vi "CR-衬丝检测处理函数.vi"(0 "Image in":T9(plugin-control), 5 "CR- 衬丝检测参数":T8={"Settings (Clamp (Rake) 1)"={"Contrast"=65, "Filter width"=3, "Steepness"=6, "Subsampling Ratio"=9, "Show Search Area"=TRUE, "Show Search Lines"=FALSE, "Show Edges Found"=FALSE, "Show Result"=TRUE}, "Options (Find Straight Edge 1)"={"Search Direction"=0, "Edge Options"={"Edge Polarity"=1, "Kernel Size"=13, "Width"=1, "Minimum Edge Strength"=25.0, "Interpolation Type"=enum."Bilinear Fixed", "Data Processing Method"=enum."Average"}, "Show Search Area"=FALSE, "Show Search Lines"=FALSE, "Show Edges Found"=FALSE, "Show Result"=FALSE, "Search Area Color"=65280, "Search Lines Color"=255, "Edge Locations Color"=16776960, "Result Color"=16711680, "Overlay Group Name"=""}, "相对距离设定"={"上限"=925.0, "下限"=3.0}, "保护套角度"={"上限"=0.0, "下限"=0.0}, "保护套直径设定"={"上限"=0.0, "下限"=0.0}, "Edge Options (Edge Detector 1)"={"Edge Polarity"=0, "Kernel Size"=3, "Width"=3, "Minimum Edge Strength"=10.0, "Interpolation Type"=enum."Bilinear Fixed", "Data Processing Method"=enum."Average"}, "保护套标准位置"={"Start X"=0, "Start Y"=0, "End X"=0, "End Y"=0}} {"保护套标准位置"."Start X" scale=0.0..1024.0; "保护套标准位置"."End X" scale=0.0..1024.0; "Edge Options (Edge Detector 1)"."Edge Polarity" items=["All Edges", "Rising Edges", "Falling Edges"]; "Options (Find Straight Edge 1)"."Search Direction" items=["Left to Right", "Right to Left", "Top to Bottom", "Bottom to Top"]; "Options (Find Straight Edge 1)"."Edge Options"."Edge Polarity" items=["All Edges", "Rising Edges", "Falling Edges"]; "Options (Find Straight Edge 1)"."Edge Options"."Minimum Edge Strength" format="%.2f"; "Options (Find Straight Edge 1)"."Edge Options"."Width" step=2; "Options (Find Straight Edge 1)"."Edge Options"."Kernel Size" step=2}, 7 "CR- 衬丝检测ROI参数":T4 {"Line 2"."Start X" scale=0.0..1024.0; "Line 2"."End X" scale=0.0..1024.0; "clamp Rectangle"."Rotation" min=-90.0 max=90.0 step=1.0 format="%.2f"; "clamp Rectangle"."Left" scale=0.0..1024.0; "clamp Rectangle"."Right" scale=0.0..1024.0; "Line 1"."Start X" scale=0.0..1024.0; "Line 1"."End X" scale=0.0..1024.0; "find straight edge Rectangle"."Rotation" min=-90.0 max=90.0 step=1.0 format="%.2f"; "find straight edge Rectangle"."Left" scale=0.0..1024.0; "find straight edge Rectangle"."Right" scale=0.0..1024.0}, 11 "error in (no error)":errorcluster caption="错误输入（无错误）") -> (4 "Image out":T9(plugin-control), 6 "Distance (Clamp (Rake) 1)":sgl format="%.2f", 8 "保护套距离":bool, 10 "衬丝有无":bool, 13 "保护套直径":sgl, 14 "保护套与基准位置差值":sgl, 15 "error out":errorcluster caption="错误输出")   [LabVIEW 2017]
uses:
  <vilib>/vision/Measure.llb/Edge Options.ctl
  <vilib>/vision/Measure.llb/Edge Polarity.ctl
  <vilib>/vision/Measure.llb/Edge New.ctl
  <vilib>/vision/NI_Vision_Development_Module.lvlib
panel:
  in  "Settings (Clamp (Rake) 1)":T1={"Contrast"=66, "Filter width"=8, "Steepness"=11, "Subsampling Ratio"=7, "Show Search Area"=TRUE, "Show Search Lines"=TRUE, "Show Edges Found"=TRUE, "Show Result"=TRUE}
  out "Angle (Real-World)":dbl
  out "保护套与基准位置差值":bool
  out "Location (Real-World)":cluster{"X":sgl, "Y":sgl}
  out "Edge Information (Edge Detector 2)":T5[](array[typedef]) {"Distance (Real-World)" format="%.2f"; "Location (Real-World)"."Y" format="%.2g"; "Location (Real-World)"."X" format="%.2f"; "Noise" format="%.2f"; "Location (Pixel)"."Y" format="%.2g"; "Location (Pixel)"."X" format="%.2f"; "Strength" format="%.2f"; "Distance (Pixel)" format="%.2f"}
  out "Edge Information (Edge Detector 1)":T5[](array[typedef]) {"Distance (Real-World)" format="%.2f"; "Location (Real-World)"."Y" format="%.2g"; "Location (Real-World)"."X" format="%.2f"; "Noise" format="%.2f"; "Location (Pixel)"."Y" format="%.2g"; "Location (Pixel)"."X" format="%.2f"; "Strength" format="%.2f"; "Distance (Pixel)" format="%.2f"}
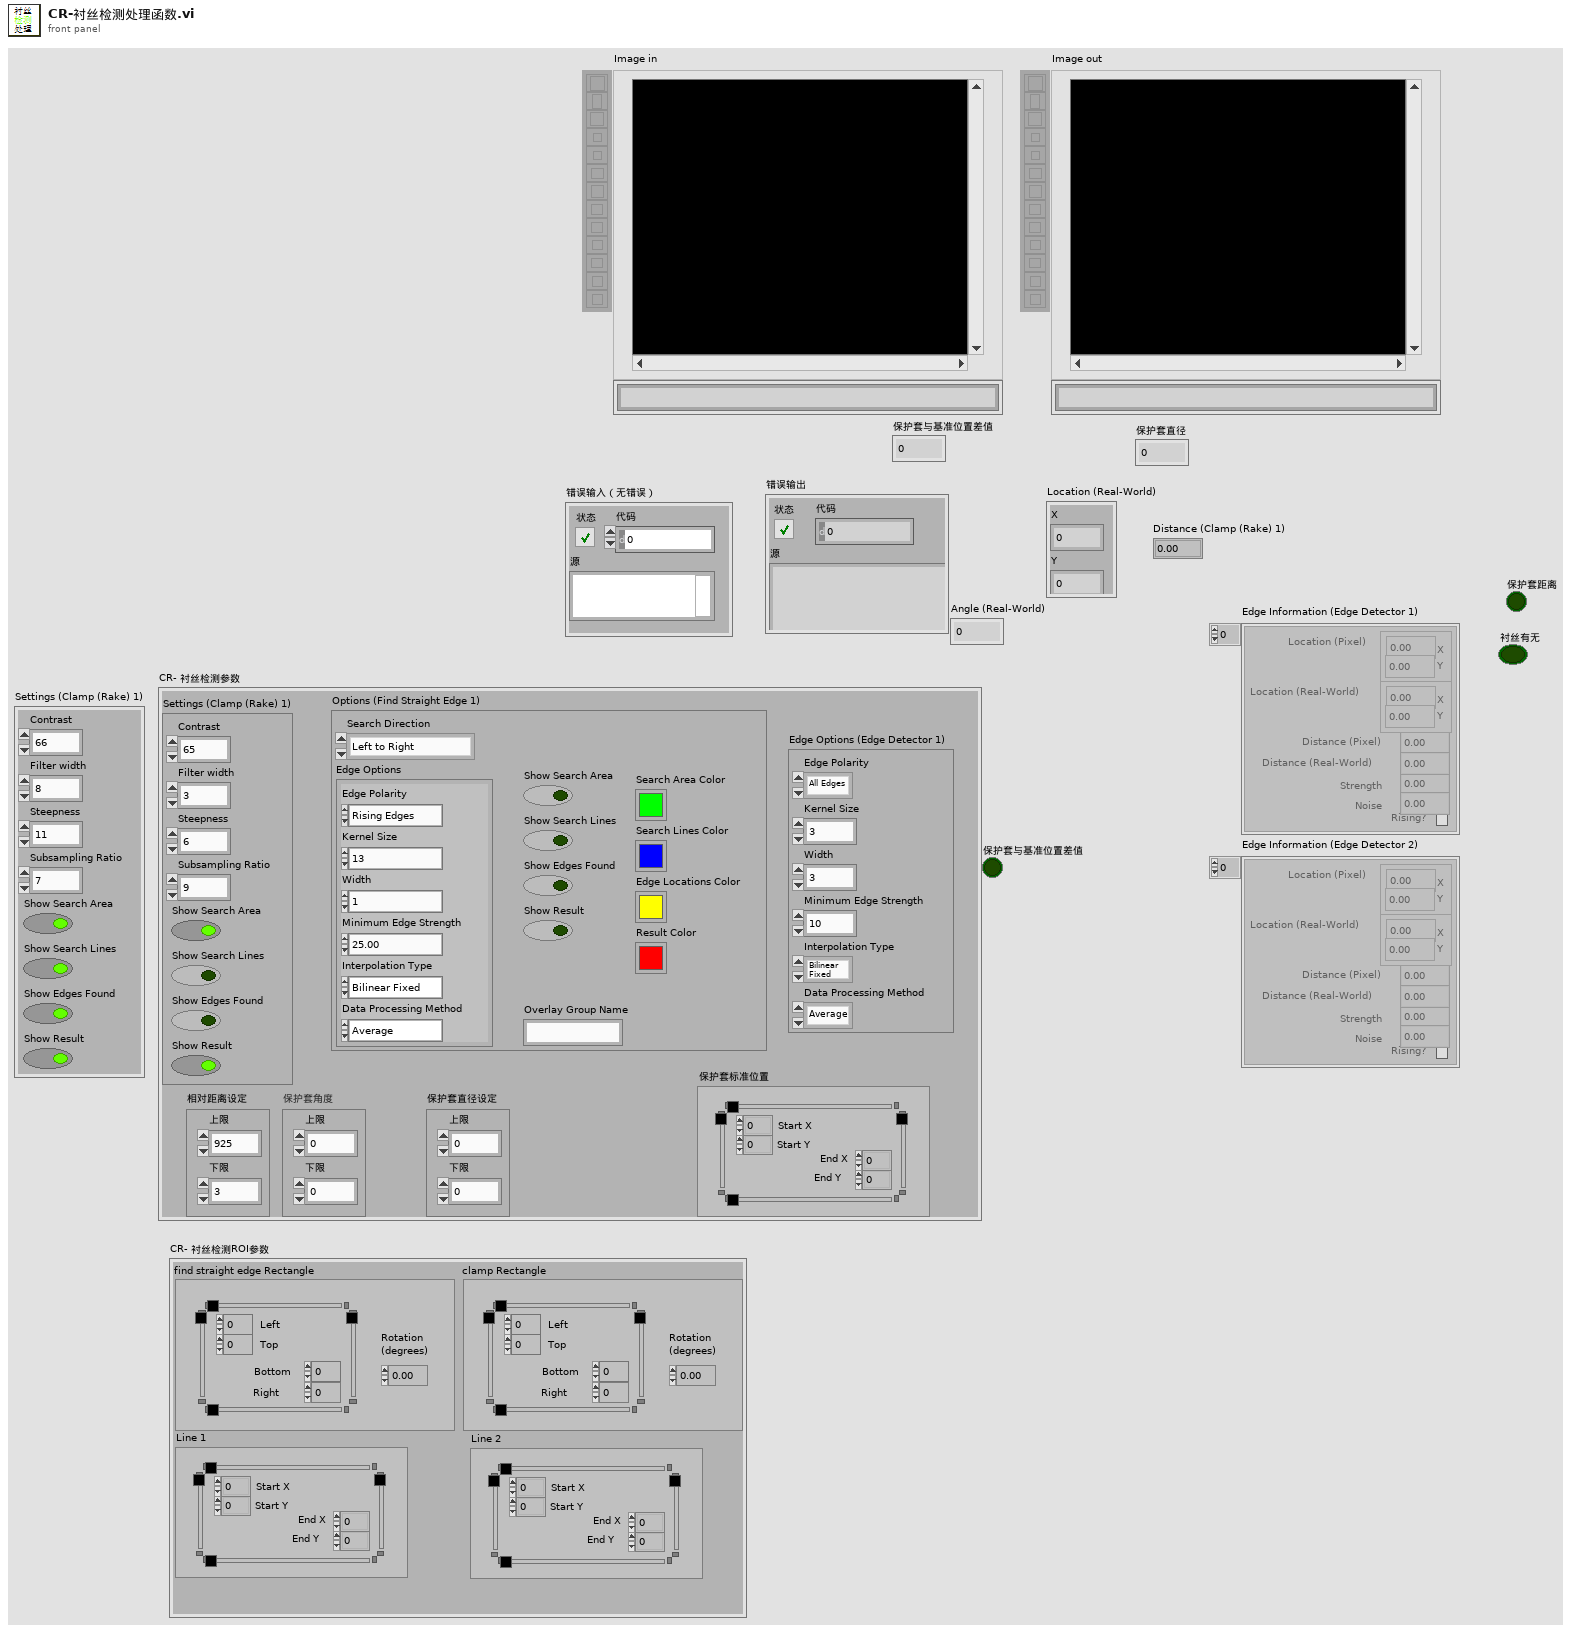
[diagram p1: front panel]
types:
  T1 = cluster{"Contrast":i32, "Filter width":i32, "Steepness":i32, "Subsampling Ratio":u32, "Show Search Area":bool, "Show Search Lines":bool, "Show Edges Found":bool, "Show Result":bool}
  T2 = typedef "IMAQ Rectangle" = cluster{"Left":i32, "Top":i32, "Right":i32, "Bottom":i32, "Rotation":dbl}
  T3 = typedef "IMAQ Line" = cluster{"Start X":i32, "Start Y":i32, "End X":i32, "End Y":i32}
  T4 = cluster{"find straight edge Rectangle":T2, "Line 1":T3, "clamp Rectangle ":T2, "Line 2":T3}
  T5 = typedef "Edge New.ctl" = cluster{"Location (Pixel)":cluster{"X":sgl, "Y":sgl}, "Location (Real-World)":cluster{"X":sgl, "Y":sgl}, "Distance (Pixel)":dbl, "Distance (Real-World)":dbl, "Strength":dbl, "Noise":dbl, "Rising?":bool}
  T6 = typedef "Edge Options.ctl" = cluster{"Edge Polarity":T7, "Kernel Size":u32, "Width":u32, "Minimum Edge Strength":sgl, "Interpolation Type":enum32{"Zero Order", "Bilinear", "Quadratic", "Cubic", "Bilinear Fixed"}, "Data Processing Method":enum32{"Average", "Median"}}
  T7 = typedef "Edge Polarity.ctl" = u32
  T8 = cluster{"Settings (Clamp (Rake) 1)":cluster{"Contrast":i32, "Filter width":i32, "Steepness":i32, "Subsampling Ratio":u32, "Show Search Area":bool, "Show Search Lines":bool, "Show Edges Found":bool, "Show Result":bool}, "Options (Find Straight Edge 1)":cluster{"Search Direction":u32, "Edge Options":T6, "Show Search Area":bool, "Show Search Lines":bool, "Show Edges Found":bool, "Show Result":bool, "Search Area Color":u32, "Search Lines Color":u32, "Edge Locations Color":u32, "Result Color":u32, "Overlay Group Name":string}, "相对距离设定":cluster{"上限":dbl, "下限":dbl}, "保护套角度":cluster{"上限":dbl, "下限":dbl}, "保护套直径设定":cluster{"上限":dbl, "下限":dbl}, "Edge Options (Edge Detector 1)":cluster{"Edge Polarity":u32, "Kernel Size":u32, "Width":u32, "Minimum Edge Strength":sgl, "Interpolation Type":enum32{"Zero Order", "Bilinear", "Quadratic", "Cubic", "Bilinear Fixed"}, "Data Processing Method":enum32{"Average", "Median"}}, "保护套标准位置":T3}
  T9 = typedef "IMAQ Image.ctl" = refnum<image>
  T10 = cluster{"Search Direction":u32, "Edge Options":T6, "Show Search Area":bool, "Show Search Lines":bool, "Show Edges Found":bool, "Show Result":bool, "Search Area Color":u32, "Search Lines Color":u32, "Edge Locations Color":u32, "Result Color":u32, "Overlay Group Name":string}
  T11 = cluster{"Global Rectangle":i32[], "Contours":cluster{"ID":enum32{"External", "Internal"}, "Type":u32, "Coordinates":i32[]}[]}
  T12 = cluster{"Desired Font (Application)":enum16{"User-specified Font", "Application Font", "System Font", "Dialog Font"}, "[User-specified Font]":cluster{"Font Name":string, "Size":i16, "Strikeout?":bool, "Italic?":bool, "Underline?":bool, "Outline?":bool, "Shadow?":bool, "Bold?":bool, "Rotation Angle":dbl}, "Horizontal Alignment":i16, "Vertical Alignment":i16}
  T13 = typedef "ROI Descriptor" = cluster{"Global Rectangle":i32[], "Contours":cluster{"ID":enum32{"External", "Internal"}, "Type":u32, "Coordinates":i32[]}[]}
  T14 = cluster{"Point1 (Pixels)":cluster{"X":sgl, "Y":sgl}, "Point2 (Pixels)":cluster{"X":sgl, "Y":sgl}, "Point1 (Real-World)":cluster{"X":sgl, "Y":sgl}, "Point2 (Real-World)":cluster{"X":sgl, "Y":sgl}, "Angle (Pixel)":dbl, "Angle (Real-World)":dbl, "Score":dbl, "Straightness":dbl, "Average SNR (db)":dbl, "Calibration Valid":bool}
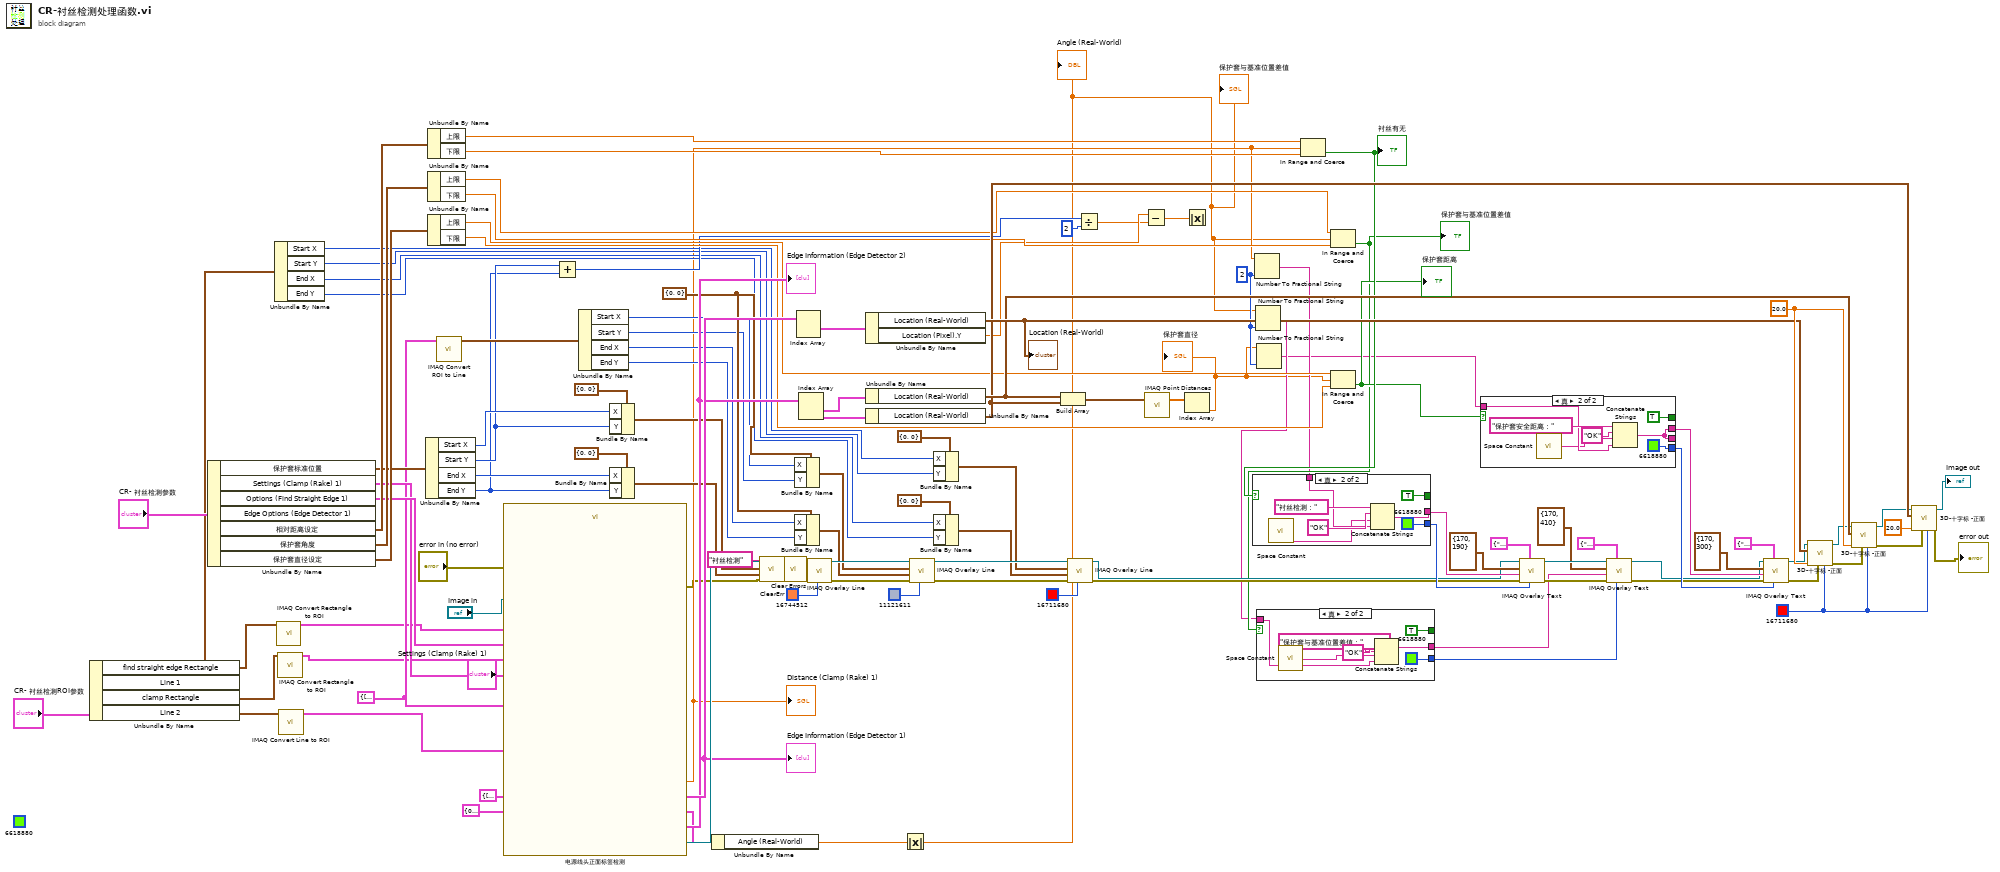
[diagram p0: block diagram]
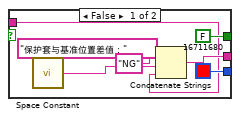
[diagram p2: hidden frame]
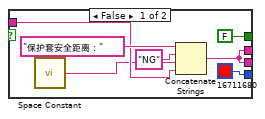
[diagram p3: hidden frame]
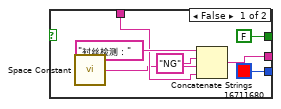
[diagram p4: hidden frame]
diagram:
  w15 = i16 2 ("精度(6)")
  w68 = cluster{"X":i32, "Y":i32} {"X"=0, "Y"=0} ("Start Point")
  w73 = T11 {"Global Rectangle"=[1263, 312, 1264, 1097], "Contours"=[{"ID"=enum."External", "Type"=2, "Coordinates"=[1263, 312, 1263, 1096]}]} ("ROI Descriptor (保护套位置)")
  (unwired) u32 6618880 ("Color")
  w105 = u32 16711680 ("Color")
  w107 = 20.0 ("radius")
  n1 = Unbundle By Name("CR- 衬丝检测ROI参数") -> ("find straight edge Rectangle"=w33:T2, "clamp Rectangle"=w32:T2, "Line 2"=w42:T3)  [unwired: 1 out]
  n2 = Unbundle By Name("CR- 衬丝检测参数") -> ("保护套标准位置"=w82:T3, "Settings (Clamp (Rake) 1)"=w84:T1, "Options (Find Straight Edge 1)"=w85:T10, "相对距离设定"=w98:cluster{"上限":dbl, "下限":dbl}, "保护套角度"=w95:cluster{"上限":dbl, "下限":dbl}, "保护套直径设定"=w94:cluster{"上限":dbl, "下限":dbl})  [unwired: 1 out]
  n3 = Unbundle By Name(w42) -> ("Start X"=w39:i32, "Start Y"=w38:i32, "End X"=w37:i32, "End Y"=w36:i32)
  n4 = call "IMAQ Convert Rectangle to ROI"("Rectangle"=w33) -> ("ROI Descriptor"=w30:T13)  [unwired: 8 in, 1 out]
  n5 = call "IMAQ Convert Rectangle to ROI"("Rectangle"=w32) -> ("ROI Descriptor"=w31:T13)  [unwired: 8 in, 1 out]
  n6 = call "IMAQ Convert Line to ROI"("Line"=w42) -> ("ROI Descriptor"=w83:T13)  [unwired: 8 in, 1 out]
  n7 = Unbundle By Name(w82) -> ("Start X"=w76:i32, "Start Y"=w60:i32, "End X"=w75:i32, "End Y"=w59:i32)
  n8 = Unbundle By Name(w98) -> ("上限"=w97:dbl, "下限"=w96:dbl)
  n9 = Unbundle By Name(w95) -> ("上限"=w93:dbl, "下限"=w92:dbl)
  n10 = Unbundle By Name(w94) -> ("上限"=w91:dbl, "下限"=w90:dbl)
  n11 = call "IMAQ Convert ROI to Line"("ROI Descriptor"=w73) -> ("Line"=w69:T3)  [unwired: 8 in, 1 out]
  n12 = call "电源线头正面标签检测"("Image In"="Image in", "ROI Descriptor (Find Straight Edge 1)"=w30, "Options (Find Straight Edge 1)"=w85, "Settings (Clamp (Rake) 1)"=w84, "ROI Descriptor (保护套位置)"=w73, "error in"="error in (no error)", "ROI Descriptor (Clamp (Rake) 1)"=w31, "ROI Descriptor (Find Straight Edge 2)"=T11 {"Global Rectangle"=[447, 110, 2174, 1857], "Contours"=[{"ID"=enum."External", "Type"=12, "Coordinates"=[447, 110, 2174, 1857, 0]}]}, "ROI Descriptor (Edge Detector 2)"=w83, "Options (Find Straight Edge 2)"=T10 {"Search Direction"=0, "Edge Options"={"Edge Polarity"=0, "Kernel Size"=3, "Width"=3, "Minimum Edge Strength"=10.0, "Interpolation Type"=enum."Bilinear Fixed", "Data Processing Method"=enum."Average"}, "Show Search Area"=FALSE, "Show Search Lines"=FALSE, "Show Edges Found"=FALSE, "Show Result"=TRUE, "Search Area Color"=65280, "Search Lines Color"=255, "Edge Locations Color"=16776960, "Result Color"=16711680, "Overlay Group Name"=""}) -> ("Image Out"=w116:T9, "Distance (Clamp (Rake) 1)"=w16:sgl, "Edge Information (保护套位置)"=w111:T5[], "Edge Information (Edge Detector 2)"=w108:T5[], "Straight Edge (Find Straight Edge 2)"=w7:T14, "error out"=w4:errorcluster)  [unwired: 11 in, 1 out]
  "Distance (Clamp (Rake) 1)" <- w16
  "Edge Information (Edge Detector 1)" <- w111
  "Edge Information (Edge Detector 2)" <- w108
  n13 = Add(x=w60, y=w59) -> (x+y=w58:i32)
  n14 = Unbundle By Name(w69) -> ("Start X"=w67:i32, "Start Y"=w66:i32, "End X"=w65:i32, "End Y"=w64:i32)
  n15 = Bundle By Name(cluster=cluster{"X":i32, "Y":i32} {"X"=0, "Y"=0} ("Start Point"), "X"=w76, "Y"=w60) -> (w78:cluster{"X":i32, "Y":i32})
  n16 = Bundle By Name(cluster=cluster{"X":i32, "Y":i32} {"X"=0, "Y"=0} ("Start Point"), "X"=w75, "Y"=w59) -> (w74:cluster{"X":i32, "Y":i32})
  n17 = Unbundle By Name(w7) -> ("Angle (Real-World)"=w6:dbl)
  n18 = call "ClearErr.vi"("error in (no error)"=w4, "运行位置"="衬丝检测") -> ("error out"=w3:errorcluster)  [unwired: 9 in]
  n19 = call <vilib>:"Clear Errors.vi"("error in (no error)"=w3) -> ("error out"=w1:errorcluster)  [unwired: 5 in, 1 out]
  n20 = Bundle By Name(cluster=w68, "X"=w67, "Y"=w66) -> (w63:cluster{"X":i32, "Y":i32})
  n21 = Bundle By Name(cluster=w68, "X"=w65, "Y"=w64) -> (w62:cluster{"X":i32, "Y":i32})
  n22 = Index Array(array=w111) -> (element #1=w110:T5)  [unwired: 2 in, 1 out]
  n23 = Index Array(array=w108) -> (element #1=w109:T5, element #2=w103:T5)  [unwired: 2 in]
  n24 = call "IMAQ Overlay Line"("Color"=u32 16744512, "error in (no error)"=w1, "End Point"=w74, "Start Point"=w78, "Image"=w116) -> ("error out"=w70:errorcluster, "Image Out"=w71:T9)  [unwired: 5 in]
  n25 = Unbundle By Name(w110) -> ("Location (Real-World)"=w106:cluster{"X":sgl, "Y":sgl}, "Location (Pixel).Y"=w61:sgl)
  "Location (Real-World)" <- w106
  n26 = Unbundle By Name(w109) -> ("Location (Real-World)"=w100:cluster{"X":sgl, "Y":sgl})
  n27 = Unbundle By Name(w103) -> ("Location (Real-World)"=w99:cluster{"X":sgl, "Y":sgl})
  n28 = Absolute Value(x=w6) -> (abs(x)=w5:dbl)
  "保护套与基准位置差值" <- w5
  "Angle (Real-World)" <- w5
  n29 = call "IMAQ Overlay Line"("Color"=u32 11121611, "error in (no error)"=w70, "End Point"=w62, "Start Point"=w63, "Image"=w71) -> ("error out"=w45:errorcluster, "Image Out"=w44:T9)  [unwired: 5 in]
  n30 = Bundle By Name(cluster=cluster{"X":i32, "Y":i32} {"X"=0, "Y"=0} ("Start Point"), "X"=w39, "Y"=w38) -> (w35:cluster{"X":i32, "Y":i32})
  n31 = Bundle By Name(cluster=cluster{"X":i32, "Y":i32} {"X"=0, "Y"=0} ("Start Point"), "X"=w37, "Y"=w36) -> (w34:cluster{"X":i32, "Y":i32})
  n32 = Build Array(w100, w99) -> (w101:cluster{"X":sgl, "Y":sgl}[])
  n33 = call "IMAQ Overlay Line"("Color"=u32 16711680, "error in (no error)"=w45, "End Point"=w34, "Start Point"=w35, "Image"=w44) -> ("error out"=w46:errorcluster, "Image Out"=w43:T9)  [unwired: 5 in]
  n34 = Divide(x=w58, y=2) -> (x/y=w56:dbl)
  n35 = Subtract(x=w61, y=w56) -> (x-y=w55:dbl)
  n36 = call "IMAQ Point Distances"("Points"=w101) -> ("Distances"=w102:sgl[])  [unwired: 4 in, 1 out]
  n37 = Absolute Value(x=w55) -> ()  [unwired: 1 out]
  n38 = Index Array(array=w102) -> (element=w12:sgl)  [unwired: 1 in]
  "保护套直径" <- w12
  n39 = Number To Fractional String(number=w16, precision (6)=w15) -> (F-format string=w14:string)  [unwired: 2 in]
  n40 = Number To Fractional String(number=w5, precision (6)=w15) -> (F-format string=w13:string)  [unwired: 2 in]
  n41 = Number To Fractional String(number=w12, precision (6)=w15) -> (F-format string=w11:string)  [unwired: 2 in]
  n42 = In Range and Coerce(upper limit=w97, x=w16, lower limit=w96) -> (In Range?=w88:bool)  [unwired: 1 out]
  "衬丝有无" <- w88
  n43 = case shown="真" w88 {
    tunnel: [FALSE TRUE] -> _
    tunnel: [u32 16711680 ("Text Color (black)") u32 6618880 ("Text Color (black)")] -> w113
    tunnel: [w120 w127] -> w112
    tunnel: w14 -> [w119 w126]
    frame False {
      n44 = call <vilib>:"Space Constant.vi"() -> ("String"=w118:string)
      n45 = Concatenate Strings("衬丝检测：", "NG" ("字符串"), w118, w119) -> (w120:string)
    }
    frame True {
      n46 = call <vilib>:"Space Constant.vi"() -> ("String"=w125:string)
      n47 = Concatenate Strings("衬丝检测：", "OK" ("字符串"), w125, w126) -> (w127:string)
    }
  }
  n48 = In Range and Coerce(upper limit=w93, x=w5, lower limit=w92) -> (In Range?=w17:bool)  [unwired: 1 out]
  "保护套与基准位置差值" <- w17
  n49 = case shown="真" w17 {
    tunnel: [FALSE TRUE] -> _
    tunnel: [u32 16711680 ("Text Color (black)") u32 6618880 ("Text Color (black)")] -> w10
    tunnel: [w134 w141] -> w18
    tunnel: w13 -> [w133 w140]
    frame False {
      n50 = call <vilib>:"Space Constant.vi"() -> ("String"=w132:string)
      n51 = Concatenate Strings("保护套与基准位置差值：", "NG" ("字符串"), w132, w133) -> (w134:string)
    }
    frame True {
      n52 = call <vilib>:"Space Constant.vi"() -> ("String"=w139:string)
      n53 = Concatenate Strings("保护套与基准位置差值：", "OK" ("字符串"), w139, w140) -> (w141:string)
    }
  }
  n54 = In Range and Coerce(upper limit=w91, x=w12, lower limit=w90) -> (In Range?=w48:bool)  [unwired: 1 out]
  "保护套距离" <- w48
  n55 = case shown="真" w48 {
    tunnel: [FALSE TRUE] -> _
    tunnel: [u32 16711680 ("Text Color (black)") u32 6618880 ("Text Color (black)")] -> w50
    tunnel: [w148 w155] -> _
    tunnel: [w148 w155] -> w49
    tunnel: w11 -> [w147 w154]
    frame False {
      n56 = call <vilib>:"Space Constant.vi"() -> ("String"=w146:string)
      n57 = Concatenate Strings("保护套安全距离：", "NG" ("字符串"), w146, w147) -> (w148:string)
    }
    frame True {
      n58 = call <vilib>:"Space Constant.vi"() -> ("String"=w153:string)
      n59 = Concatenate Strings("保护套安全距离：", "OK" ("字符串"), w153, w154) -> (w155:string)
    }
  }
  n60 = call "IMAQ Overlay Text"("Text Color (black)"=w113, "Font, Size & Style"=T12 {"Desired Font (Application)"=enum."User-specified Font", "[User-specified Font]"={"Font Name"="", "Size"=100, "Strikeout?"=FALSE, "Italic?"=FALSE, "Underline?"=FALSE, "Outline?"=FALSE, "Shadow?"=FALSE, "Bold?"=FALSE, "Rotation Angle"=0.0}, "Horizontal Alignment"=0, "Vertical Alignment"=0}, "error in (no error)"=w46, "String"=w112, "Origin"=cluster{"X":i32, "Y":i32} {"X"=170, "Y"=190}, "Image"=w43) -> ("error out"=w22:errorcluster, "Image Out"=w20:T9)  [unwired: 4 in]
  n61 = call "IMAQ Overlay Text"("Text Color (black)"=w10, "Font, Size & Style"=T12 {"Desired Font (Application)"=enum."User-specified Font", "[User-specified Font]"={"Font Name"="", "Size"=100, "Strikeout?"=FALSE, "Italic?"=FALSE, "Underline?"=FALSE, "Outline?"=FALSE, "Shadow?"=FALSE, "Bold?"=FALSE, "Rotation Angle"=0.0}, "Horizontal Alignment"=0, "Vertical Alignment"=0}, "error in (no error)"=w22, "String"=w18, "Origin"=cluster{"X":i32, "Y":i32} {"X"=170, "Y"=410}, "Image"=w20) -> ("error out"=w23:errorcluster, "Image Out"=w21:T9)  [unwired: 4 in]
  n62 = call "IMAQ Overlay Text"("Text Color (black)"=w50, "Font, Size & Style"=T12 {"Desired Font (Application)"=enum."User-specified Font", "[User-specified Font]"={"Font Name"="", "Size"=100, "Strikeout?"=FALSE, "Italic?"=FALSE, "Underline?"=FALSE, "Outline?"=FALSE, "Shadow?"=FALSE, "Bold?"=FALSE, "Rotation Angle"=0.0}, "Horizontal Alignment"=0, "Vertical Alignment"=0}, "error in (no error)"=w23, "String"=w49, "Origin"=cluster{"X":i32, "Y":i32} {"X"=170, "Y"=300}, "Image"=w21) -> ("error out"=w51:errorcluster, "Image Out"=w52:T9)  [unwired: 4 in]
  n63 = call "3D-十字标 -正面.vi"("Color"=w105, "error in (no error)"=w51, "radius"=w107, "Target Point"=w106, "输入图片"=w52) -> ("error out"=w28:errorcluster, "输出图片"=w29:T9)  [unwired: 5 in]
  n64 = call "3D-十字标 -正面.vi"("Color"=w105, "error in (no error)"=w28, "radius"=w107, "Target Point"=w100, "输入图片"=w29) -> ("error out"=w25:errorcluster, "输出图片"=w26:T9)  [unwired: 5 in]
  n65 = call "3D-十字标 -正面.vi"("Color"=w105, "error in (no error)"=w25, "radius"=20.0, "Target Point"=w99, "输入图片"=w26) -> ("error out"=→"error out":errorcluster, "输出图片"=→"Image out":T9)  [unwired: 5 in]
